vi "Set Acquisition Config Analog In.vi"(7 "AcqMode":T1, 8 "error in (no error)":errorcluster, 9 "nSize":i32, 10 "hzFrquency":dbl, 11 "hdwf":i32) -> (0 "error out":errorcluster, 1 "function return":i32, 3 "hdwf out":i32)   [LabVIEW 2012, in "AnalogDiscSDKLv.lvlib"]
doc: "extern \"C\" __declspec(dllexport) int SetAcquisitionConfig_AnalogIn(HDWF hdwf,\n double hzFrquency, int nSize, ACQMODE AcqMode );"
uses:
  <instrlib>/AnalogDiscSDKLv/AnalogDiscSDKLv.lvlib
  <instrlib>/AnalogDiscSDKLv/VIs/DWF_AcqMode.ctl
  <instrlib>/AnalogDiscSDKLv/AnalogDiscSDKLv.dll
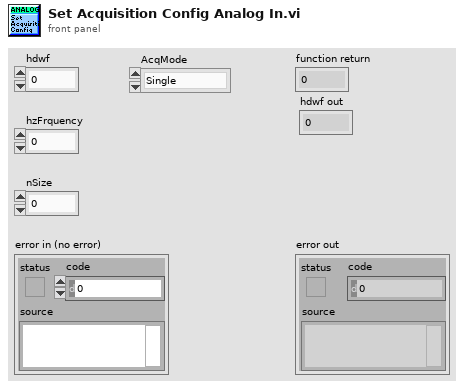
[diagram p1: front panel]
types:
  T1 = typedef "DWF_AcqMode.ctl" = enum16{"Single", "ScanShift", "ScanScreen", "Record"}
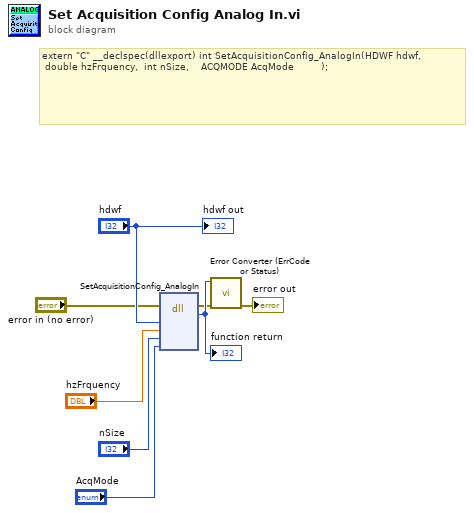
[diagram p0: block diagram]
diagram:
  # "extern \"C\" __declspec(dllexport) int SetAcquisitionConfig_AnalogIn(HDWF hdwf,\n\tdouble hzFrquency,\t\tint nSize,\t\t\t\tACQMODE AcqMode\t\t\t\t\t\t\t\t\t);"
  n1 = dll-call lib="C:/Program Files (x86)/National Instruments/LabVIEW 2012/instr.lib/AnalogDiscSDKLv/AnalogDiscSDKLv.*" fn="SetAcquisitionConfig_AnalogIn"(error in="error in (no error)", "hdwf"="hdwf", "hzFrquency"="hzFrquency", "nSize"="nSize", "AcqMode"="AcqMode") -> (error out=w2:errorcluster, w8:i32)  [unwired: 6 in, 1 out]
  "function return" <- w8
  n2 = call <instrlib>:"Error Converter (ErrCode or Status).vi"("error in (no error)"=w2, "error code"=w8) -> ("error out"=→"error out":errorcluster)  [unwired: 9 in]
  "hdwf out" <- "hdwf"
